vi "WaveformForm.vi"(10 "Data":dbl[][](array[numeric]), 11 "dt":dbl) -> (3 "WaveformData":waveform(dbl)[](array[waveform]))   [LabVIEW 2019]
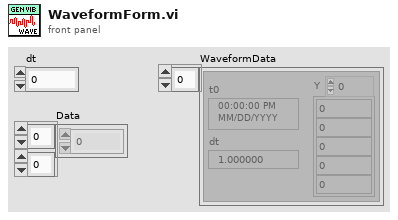
[diagram p1: front panel]
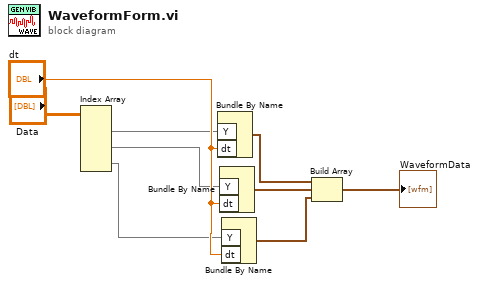
[diagram p0: block diagram]
diagram:
  n1 = Index Array(array="Data") -> (element #1=w2:dbl[], element #2=w3:dbl[], element #3=w4:dbl[])  [unwired: 6 in]
  n2 = Bundle By Name("Y"=w2, "dt"="dt") -> (w6:waveform(dbl))  [unwired: 1 in]
  n3 = Bundle By Name("Y"=w3, "dt"="dt") -> (w7:waveform(dbl))  [unwired: 1 in]
  n4 = Bundle By Name("Y"=w4, "dt"="dt") -> (w8:waveform(dbl))  [unwired: 1 in]
  n5 = Build Array(w6, w7, w8) -> (→"WaveformData":waveform(dbl)[])
